vi "Ismatec ISM831C Test Program.vi"() -> ()   [LabVIEW 2018, in "Ismatec ISM 831C.lvlib"]
uses:
  Ismatec ISM 831C.lvlib
  Controls/Ismatech ISM831C Settings Cluster.ctl
panel:
  in  "stop":bool
  out "Connection Error 2":bool
  out "Pump On?":enum16{"Off", "On", "Not Initialized"}(ring)
  out "Connection Error":bool
  in  "Speed (%)":dbl
  out "error out":errorcluster
  in  "error in (no error)":errorcluster
  out "Ismatech Settings":T1={"VISA resource name"="", "Simulated?"=TRUE, "Pump Number"=1.0, "Reverse?"=FALSE} {"Pump Number" min=1.0 max=20.0 step=1.0}
  in  "Ismatech Settings":T1={"VISA resource name"="", "Simulated?"=TRUE, "Pump Number"=1.0, "Reverse?"=FALSE} {"Pump Number" min=1.0 max=20.0 step=1.0}
  in  "Pause":bool
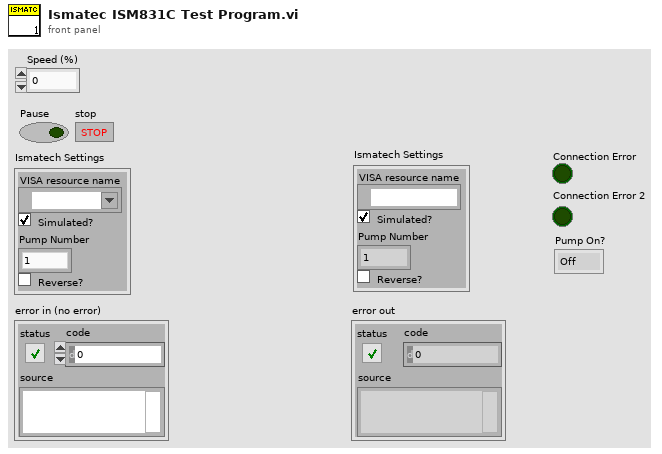
[diagram p1: front panel]
types:
  T1 = typedef "Ismatec ISM 831C.lvlib/Ismatech ISM831C Settings Cluster.ctl" = cluster{"VISA resource name":refnum<visa-resource-name>, "Simulated?":bool, "Pump Number":dbl, "Reverse?":bool}
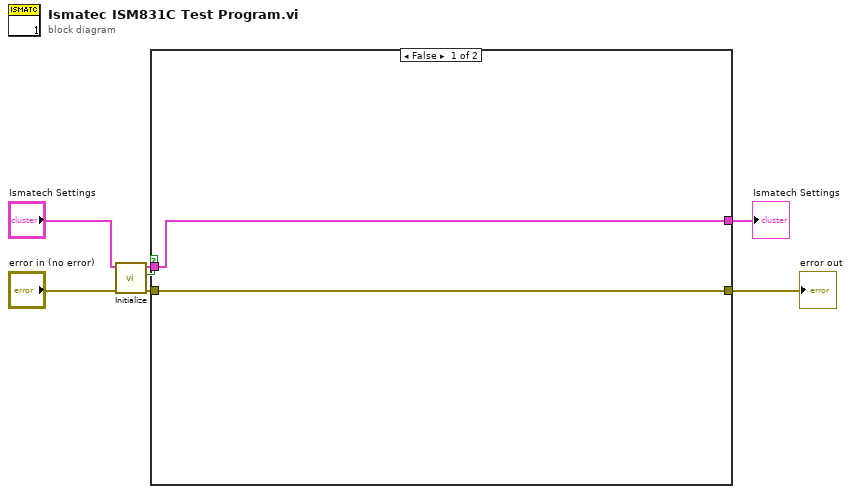
[diagram p0: block diagram]
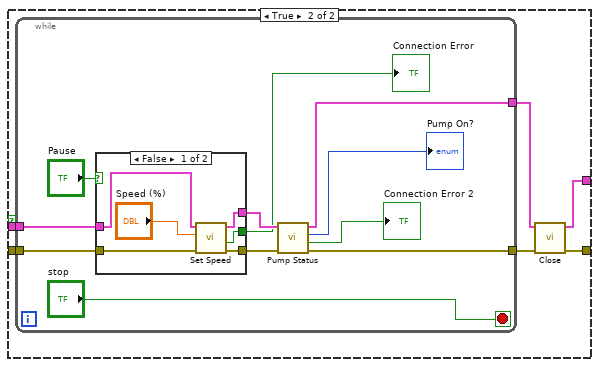
[diagram p2: hidden frame]
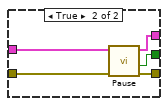
[diagram p3: hidden frame]
diagram:
  n1 = call "Initialize.vi"("error in (no error)"="error in (no error)", "Ismatech Settings"="Ismatech Settings") -> ("error out"=w4:errorcluster, "No Pump Connected"=w1:bool, "Ismatech Settings"=w5:T1)  [unwired: 6 in, 1 out]
  n2 = case shown="False" w1 {
    tunnel: w5 -> [w9 w15]
    tunnel: w4 -> [w8 w14]
    tunnel: [w9 w12] -> w3
    tunnel: [w8 w10] -> w2
    frame False {
    }
    frame True {
      n3 = while {
        tunnel: w15 -> [w25]
        tunnel: w14 -> [w24]
        tunnel: [w21] -> w13
        tunnel: [w20] -> w11
        stop <- "stop" stop-if-true
        n4 = case shown="False" "Pause" {
          tunnel: w25 -> [w32 w37]
          tunnel: w24 -> [w31 w36]
          tunnel: [w29 w35] -> w23
          tunnel: [w28 w34] -> w22
          tunnel: [w27 w33] -> w19
          frame False {
            n5 = call "Set Speed.vi"("error in (no error)"=w31, "Speed (%)"="Speed (%)", "Ismatech Settings In"=w32) -> ("error out"=w28:errorcluster, "Connection Error"=w27:bool, "Ismatech Settings Out"=w29:T1)  [unwired: 6 in]
          }
          frame True {
            n6 = call "Pause.vi"("error in (no error)"=w36, "Ismatech Settings In"=w37) -> ("error out"=w34:errorcluster, "Connection Error"=w33:bool, "Ismatech Settings Out"=w35:T1)  [unwired: 7 in]
          }
        }
        "Connection Error" <- w19
        n7 = call "Pump Status.vi"("error in (no error)"=w22, "Ismatech Settings In"=w23) -> ("error out"=w20:errorcluster, "Connection Error"=→"Connection Error 2":bool, "Pump On?"=→"Pump On?":enum16{"Off", "On", "Not Initialized"}, "Ismatech Settings Out"=w21:T1)  [unwired: 6 in]
      }
      n8 = call "Close.vi"("error in (no error)"=w11, "Ismatech Settings"=w13) -> ("error out"=w10:errorcluster, "Ismatech Settings"=w12:T1)  [unwired: 7 in, 1 out]
    }
  }
  "Ismatech Settings" <- w3
  "error out" <- w2
